vi "TEST Object Manual Bounds (Non Default Scaling Offset).vi"() -> ()   [LabVIEW 2021, in "IObject.lvclass"]
uses:
  IObject.lvclass
  <vilib>/Utility/miscctls.llb/LVRectTypeDef.ctl
  Object/Object.lvclass
panel:
  in  "OK Button 2":bool
  in  "Bounds":T1={"Left"=100, "Top"=60, "Right"=410, "Bottom"=260}
  in  "OK Button 1":bool
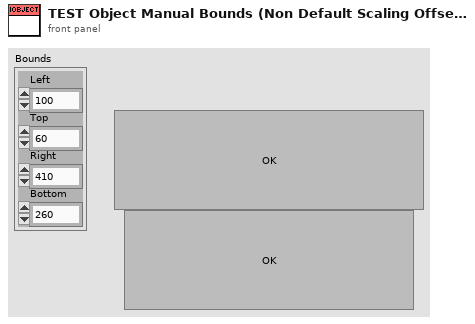
[diagram p1: front panel]
types:
  T1 = typedef "LVRectTypeDef.ctl" = cluster{"Left":i16, "Top":i16, "Right":i16, "Bottom":i16}
  T2 = cluster{"Left":dbl, "Top":dbl, "Right":dbl, "Bottom":dbl}[]
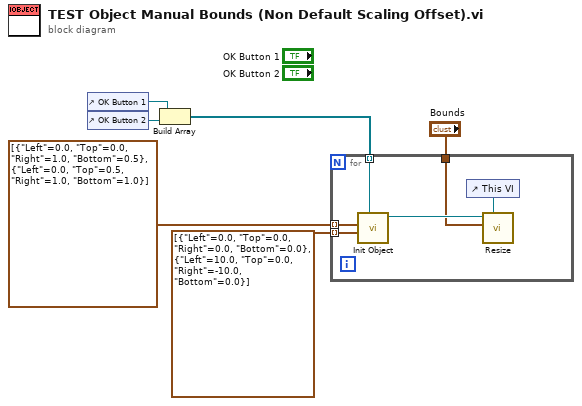
[diagram p0: block diagram]
diagram:
  n1 = control-ref of="OK Button 1"() -> (w6:refnum<vi>)
  n2 = control-ref of="OK Button 2"() -> (w5:refnum<vi>)
  n3 = Build Array(w6, w5) -> (w4:refnum<vi>[])
  n4 = for {
    tunnel: T2 [{"Left"=0.0, "Top"=0.0, "Right"=1.0, "Bottom"=0.5}, {"Left"=0.0, "Top"=0.5, "Right"=1.0, "Bottom"=1.0}] -> [w10] mode=indexing
    tunnel: w4 -> [w9] mode=indexing
    tunnel: "Bounds" -> [w8]
    tunnel: T2 [{"Left"=0.0, "Top"=0.0, "Right"=0.0, "Bottom"=0.0}, {"Left"=10.0, "Top"=0.0, "Right"=-10.0, "Bottom"=0.0}] -> [w7] mode=indexing
    n5 = call "Init Object.vi"("GObj Refnum"=w9, "B [0, 0, 0, 0]"=w7, "A [0, 0, 1, 1]"=w10) -> ("MMI Scaling out"=w12:refnum<class "Object.lvclass">)  [unwired: 7 in, 1 out]
    n6 = control-ref of="This VI"() -> (w11:refnum<vi>)
    n7 = call-dynamic "Resize.vi"("VI Refnum"=w11, "Bounds"=w8, "MMI Scaling in"=w12) -> ()  [unwired: 6 in, 3 out]
  }
